vi "protocol.vi"() -> ()   [LabVIEW 2016]
uses:
  <vilib>/Instr/_visa.llb/VISA Configure Serial Port (Instr).vi
panel:
  out "vel rotation":u8[](array[numeric])
  out "vel normal":u8[](array[numeric])
  out "vel radial":u8[](array[numeric])
  in  "stop":bool
  out "return count":u32
  out "error out":errorcluster
  in  "termination char\n(0xA = '\\n' = LF)":u8=10 format="%.0x"
  in  "VISA resource name":refnum<visa-resource-name>
  in  "Serial Settings":T1={"baud rate"=9600, "data bits"=8, "parity"=enum."None", "stop bits"=10, "flow control"=0} {"flow control" items=["None"=0, "XON/XOFF"=1, "RTS/CTS"=2, "DTR/DSR"=4]; "stop bits" items=["1.0"=10, "1.5"=15, "2.0"=20]; "data bits" min=5 max=8 step=1; "baud rate" items=["75"=75, "110"=110, "134"=134, "150"=150, "300"=300, "600"=600, "1200"=1200, "1800"=1800, "2400"=2400, "4800"=4800, "7200"=7200, "9600"=9600, "14400"=14400, "19200"=19200, "28800"=28800, "38400"=38400, "56000"=56000, "57600"=57600, "115200"=115200, "128000"=128000, "230400"=230400]}
  in  "vel radial":i16
  in  "vel normal":i16
  in  "vel rotation":i16
  in  "pos 3":i16=3468
  in  "pos 2":i16=3468
  in  "pos 1":i16=3468
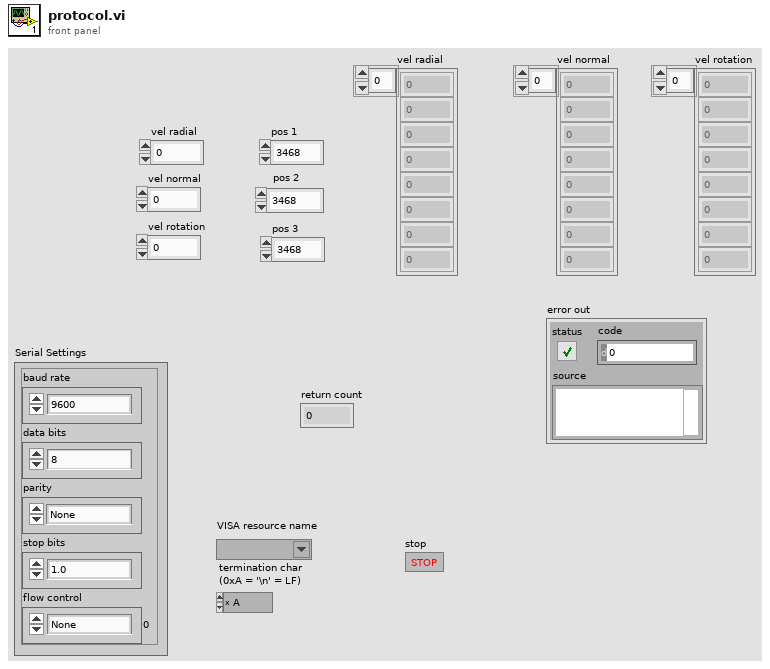
[diagram p1: front panel]
types:
  T1 = cluster{"baud rate":u32, "data bits":u16, "parity":enum16{"None", "Odd", "Even", "Mark", "Space"}, "stop bits":u16, "flow control":u16}
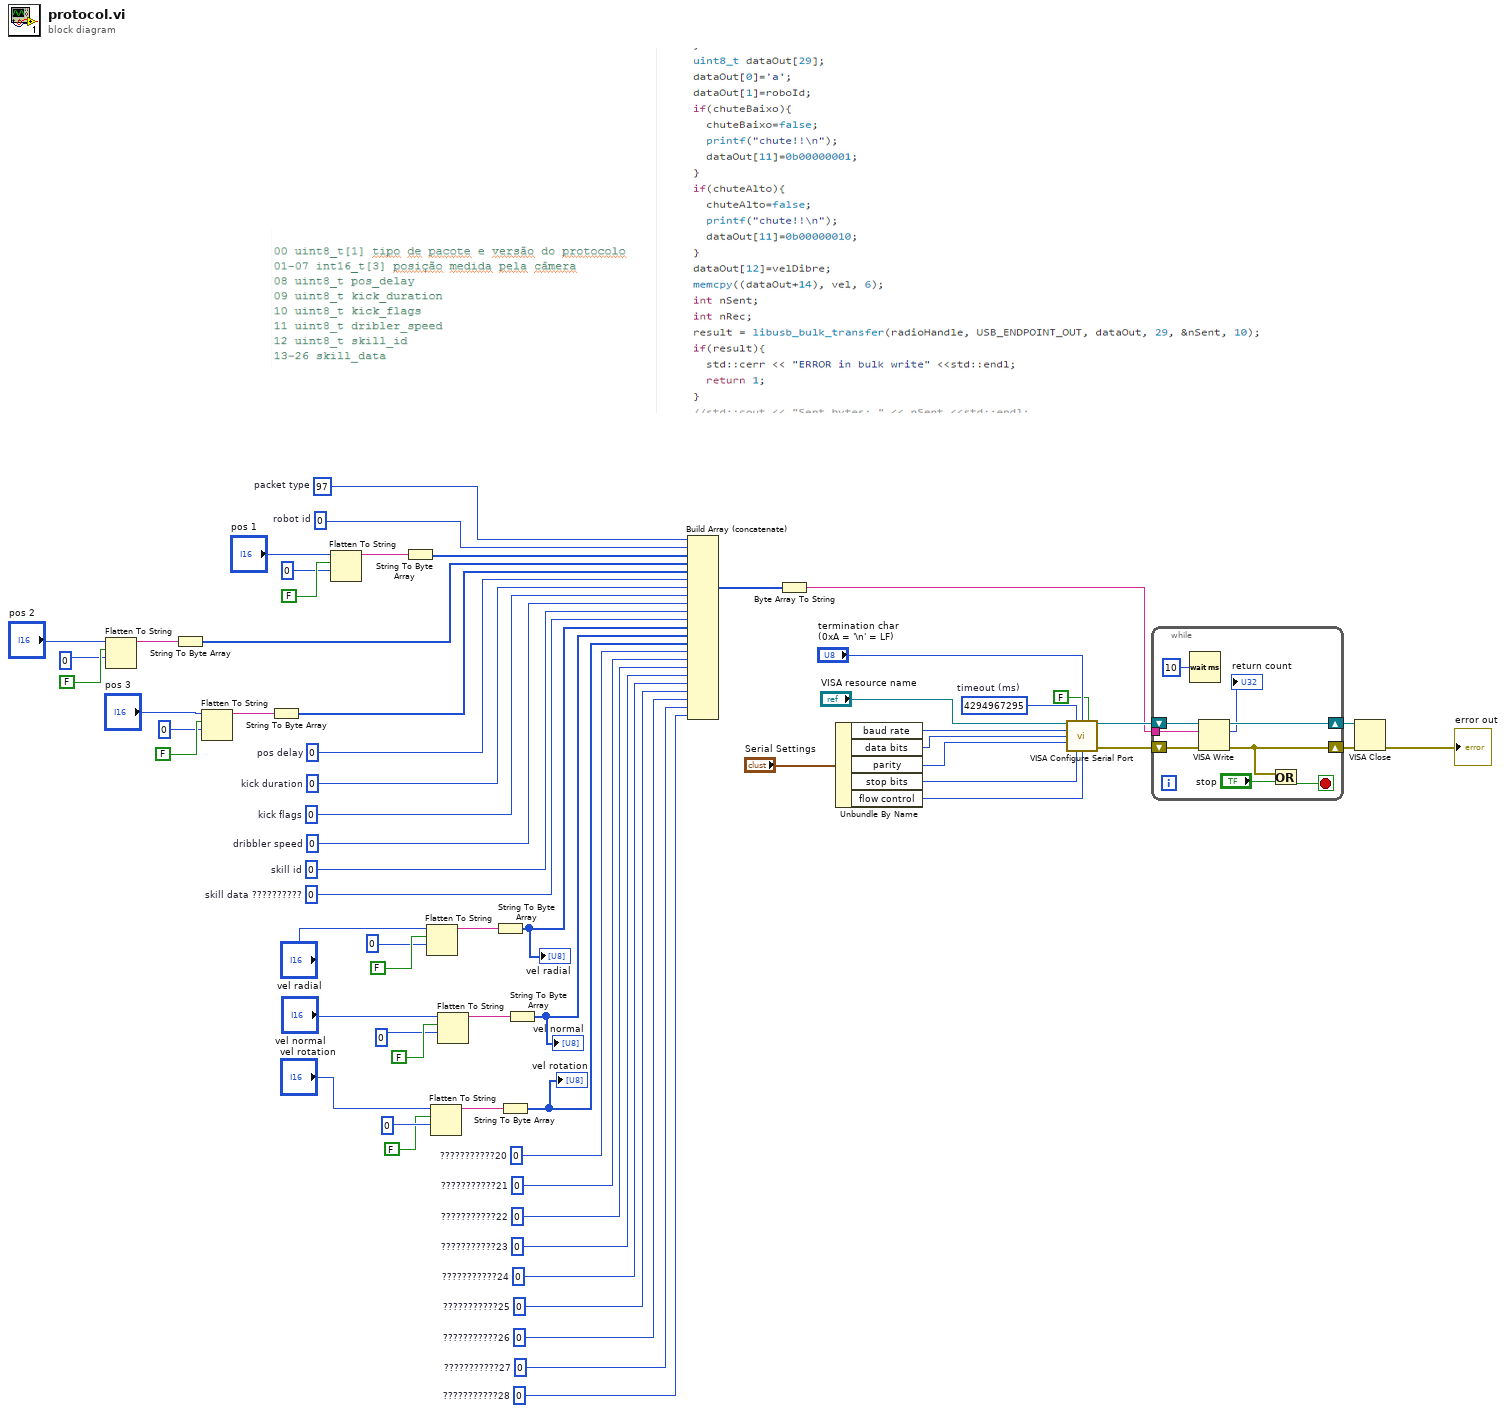
[diagram p0: block diagram]
diagram:
  w1 = u32 4294967295  # timeout (ms)
  w2 = u8 0  # skill data ??????????
  w6 = u8 0  # ???????????28
  w7 = u8 0  # ???????????27
  w8 = u8 0  # ???????????26
  w10 = u8 0  # ???????????25
  w9 = u8 0  # ???????????24
  w11 = u8 0  # ???????????23
  w12 = u8 0  # ???????????22
  w13 = u8 0  # ???????????21
  w14 = u8 0  # ???????????20
  w37 = u8 0  # skill id
  w63 = u8 0  # dribbler speed
  w32 = u8 0  # kick flags
  w38 = u8 0  # kick duration
  w39 = u8 0  # pos delay
  w34 = u8 0  # robot id
  w64 = u8 97  # packet type
  n1 = Flatten To String(anything="pos 2", prepend array or string size? (T)=FALSE, byte order (0:big-endian, network order)=u16 0) -> (data string=w55:string)  [unwired: 1 in, 2 out]
  n2 = String To Byte Array(string=w55) -> (unsigned byte array=w33:u8[])
  n3 = Flatten To String(anything="pos 3", prepend array or string size? (T)=FALSE, byte order (0:big-endian, network order)=u16 0) -> (data string=w51:string)  [unwired: 1 in, 2 out]
  n4 = String To Byte Array(string=w51) -> (unsigned byte array=w49:u8[])
  n5 = Flatten To String(anything="pos 1", prepend array or string size? (T)=FALSE, byte order (0:big-endian, network order)=u16 0) -> (data string=w60:string)  [unwired: 1 in, 2 out]
  n6 = String To Byte Array(string=w60) -> (unsigned byte array=w59:u8[])
  n7 = Flatten To String(anything="vel radial", prepend array or string size? (T)=FALSE, byte order (0:big-endian, network order)=u16 0) -> (data string=w46:string)  [unwired: 1 in, 2 out]
  n8 = Flatten To String(anything="vel rotation", prepend array or string size? (T)=FALSE, byte order (0:big-endian, network order)=u16 0) -> (data string=w41:string)  [unwired: 1 in, 2 out]
  n9 = Flatten To String(anything="vel normal", prepend array or string size? (T)=FALSE, byte order (0:big-endian, network order)=u16 0) -> (data string=w42:string)  [unwired: 1 in, 2 out]
  n10 = String To Byte Array(string=w46) -> (unsigned byte array=w5:u8[])
  "vel radial" <- w5
  n11 = String To Byte Array(string=w41) -> (unsigned byte array=w3:u8[])
  "vel rotation" <- w3
  n12 = String To Byte Array(string=w42) -> (unsigned byte array=w4:u8[])
  "vel normal" <- w4
  n13 = Build Array (concatenate)(w64, w34, w59, w33, w49, w39, w38, w32, w63, w37, w2, w5, w4, w3, w14, w13, w12, w11, w9, w10, w8, w7, w6) -> (w16:u8[])
  n14 = Byte Array To String(unsigned byte array=w16) -> (string=w15:string)
  n15 = Unbundle By Name("Serial Settings") -> ("baud rate"=w29:u32, "data bits"=w28:u16, "parity"=w27:enum16{"None", "Odd", "Even", "Mark", "Space"}, "stop bits"=w26:u16, "flow control"=w25:u16)
  n16 = call-poly "VISA Configure Serial Port"("VISA resource name"="VISA resource name", "timeout (10sec)"=w1, "termination char\n(0xA = '\\n' = LF)"="termination char\n(0xA = '\\n' = LF)", "Enable Termination\nChar (T)"=FALSE ("Enable Termination\nChar (T)"), "baud rate (9600)"=w29, "data bits (8)"=w28, "parity (0:none)"=w27, "stop bits (10: 1 bit)"=w26, "flow control (0:none)"=w25) -> ("VISA resource name out"=w21:refnum<visa-resource-name>, "error out"=w19:errorcluster)  [unwired: 5 in]
  n17 = while {
    tunnel: w15 -> [w70]
    shift-right: [w72] -> w20
    shift-left: w21 -> [w73]
    shift-right: [w66] -> w18
    shift-left: w19 -> [w71]
    stop <- w67 stop-if-true
    n18 = Wait (ms)(milliseconds to wait=u32 10) -> ()  [unwired: 1 out]
    n19 = VISA Write(VISA resource name=w73, write buffer=w70, error in (no error)=w71) -> (VISA resource name out=w72:refnum<visa-resource-name>, return count=→"return count":u32, error out=w66:errorcluster)
    n20 = Or(x=w66, y="stop") -> (x .or. y?=w67:bool)
  }
  n21 = VISA Close(VISA resource name=w20, error in (no error)=w18) -> (error out=→"error out":errorcluster)
